vi "dynamic_calc.vi"(7 "index (row)":i32, 8 "error constant":errorcluster, 9 "DYNAMIC":T1(array[cluster]), 10 "Array 2":T2(array[cluster]), 11 "x  dist":dbl[](array[numeric])=[77911.0, 79996.0, 60540.0, 54460.0, 36220.0]) -> (0 "error constant 2":errorcluster, 2 "time":dbl[](array[numeric]), 3 "Array":dbl[](array[numeric]))   [LabVIEW 2015]
panel:
  out "number":dbl[](array[numeric])
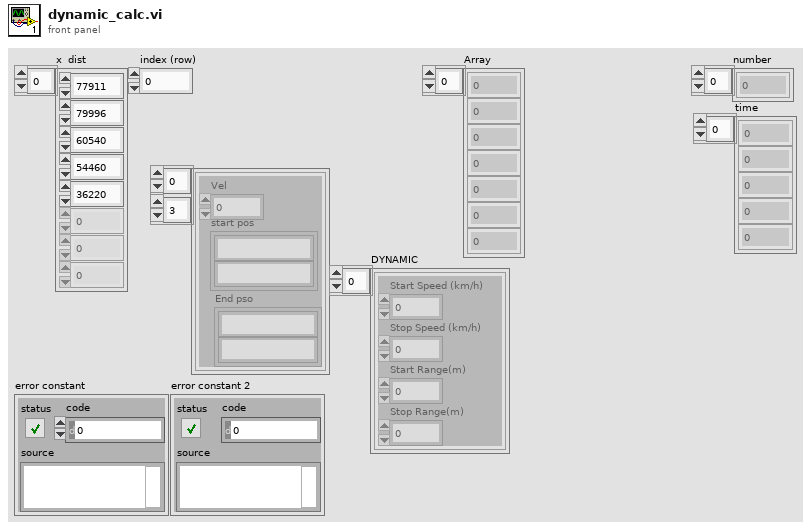
[diagram p1: front panel]
types:
  T1 = cluster{"Start Speed (km/h)":dbl, "Stop Speed (km/h) ":dbl, "Start Range(m)":dbl, "Stop Range(m)":dbl}[]
  T2 = cluster{"Vel":dbl, "start pos":cluster{string, string}, "End pso":cluster{string, string}}[][]
  T3 = cluster{"Vel":dbl, "start pos":cluster{string, string}, "End pso":cluster{string, string}}[]
  T4 = cluster{"Start Speed (km/h)":dbl, "Stop Speed (km/h) ":dbl, "Start Range(m)":dbl, "Stop Range(m)":dbl}
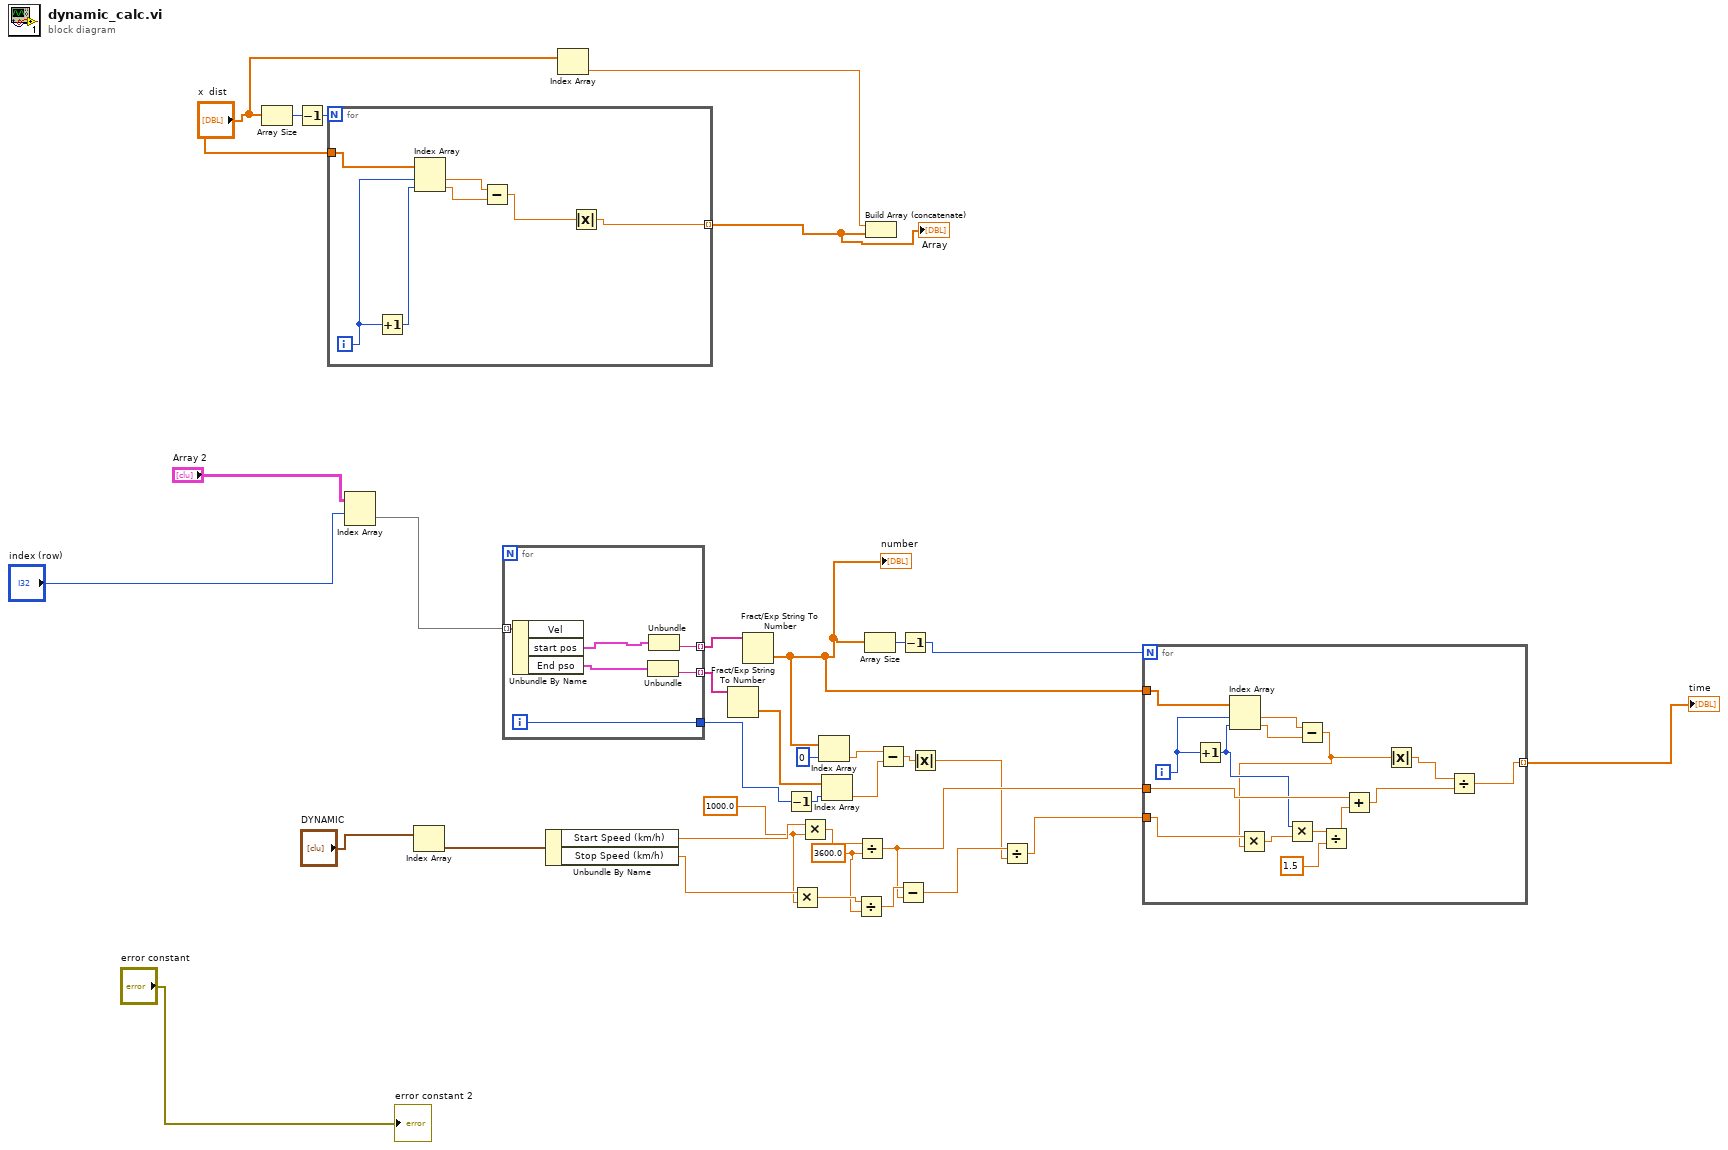
[diagram p0: block diagram]
diagram:
  w15 = 3600.0 ("y")
  w17 = 1000.0 ("y")
  n1 = Array Size(array="x  dist") -> (size(s)=w34:i32)
  n2 = Decrement(x=w34) -> (x-1=w35:i32)
  n3 = for {
    N: w35 -> [_]
    tunnel: "x  dist" -> [w42]
    tunnel: [w36] -> w26 mode=indexing
    i -> [w40]
    n4 = Increment(x=w40) -> (x+1=w41:i32)
    n5 = Index Array(array=w42, index #1=w40, index #2=w41) -> (element #1=w39:dbl, element #2=w38:dbl)
    n6 = Subtract(x=w39, y=w38) -> (x-y=w37:dbl)
    n7 = Absolute Value(x=w37) -> (abs(x)=w36:dbl)
  }
  "Array" <- w26
  n8 = Index Array(array="Array 2", index (row)="index (row)") -> (element=w30:T3)  [unwired: 1 in]
  n9 = Index Array(array="DYNAMIC") -> (element=w23:T4)  [unwired: 1 in]
  n10 = for {
    tunnel: w30 -> [w48] mode=indexing
    tunnel: [w46] -> w29 mode=indexing
    tunnel: [w44] -> w20 mode=indexing
    tunnel: [w43] -> w1
    i -> [w43]
    n11 = Unbundle By Name(w48) -> ("start pos"=w47:cluster{string, string}, "End pso"=w45:cluster{string, string})  [unwired: 1 out]
    n12 = Unbundle(w45) -> (w44:string)  [unwired: 1 out]
    n13 = Unbundle(w47) -> (w46:string)  [unwired: 1 out]
  }
  n14 = Unbundle By Name(w23) -> ("Start Speed (km/h)"=w19:dbl, "Stop Speed (km/h)"=w18:dbl)
  n15 = Index Array(array="x  dist") -> (element=w32:dbl)  [unwired: 1 in]
  n16 = Fract/Exp String To Number(string=w20) -> (number=w8:dbl[])  [unwired: 3 in, 1 out]
  n17 = Fract/Exp String To Number(string=w29) -> (number=w9:dbl[])  [unwired: 3 in, 1 out]
  "number" <- w9
  n18 = Decrement(x=w1) -> (x-1=w2:i32)
  n19 = Multiply(x=w18, y=w17) -> (x*y=w16:dbl)
  n20 = Multiply(x=w19, y=w17) -> (x*y=w24:dbl)
  n21 = Index Array(array=w9, index=0) -> (element=w5:dbl)
  n22 = Index Array(array=w8, index=w2) -> (element=w6:dbl)
  n23 = Divide(x=w16, y=w15) -> (x/y=w11:dbl)
  n24 = Divide(x=w24, y=w15) -> (x/y=w10:dbl)
  n25 = Array Size(array=w9) -> (size(s)=w28:i32)
  n26 = Build Array (concatenate)(w32, w26) -> ()  [unwired: 1 out]
  n27 = Subtract(x=w5, y=w6) -> (x-y=w4:dbl)
  n28 = Subtract(x=w11, y=w10) -> (x-y=w13:dbl)
  n29 = Decrement(x=w28) -> (x-1=w27:i32)
  n30 = Absolute Value(x=w4) -> (abs(x)=w3:dbl)
  n31 = Divide(x=w13, y=w3) -> (x/y=w12:dbl)
  n32 = for {
    N: w27 -> [_]
    tunnel: w9 -> [w63]
    tunnel: [w58] -> w25 mode=indexing
    tunnel: w10 -> [w57]
    tunnel: w12 -> [w51]
    i -> [w62]
    n33 = Increment(x=w62) -> (x+1=w56:i32)
    n34 = Index Array(array=w63, index #1=w62, index #2=w56) -> (element #1=w61:dbl, element #2=w60:dbl)
    n35 = Subtract(x=w61, y=w60) -> (x-y=w50:dbl)
    n36 = Multiply(x=w51, y=w50) -> (x*y=w49:dbl)
    n37 = Multiply(x=w56, y=w49) -> (x*y=w55:dbl)
    n38 = Divide(x=w55, y=1.5) -> (x/y=w53:dbl)
    n39 = Add(x=w57, y=w53) -> (x+y=w52:dbl)
    n40 = Absolute Value(x=w50) -> (abs(x)=w59:dbl)
    n41 = Divide(x=w59, y=w52) -> (x/y=w58:dbl)
  }
  "time" <- w25
  "error constant 2" <- "error constant"
